vi "Read Mode Command.vi"   [LabVIEW 2023, in "Control Mode.lvclass"]
uses:
  Control Mode.lvclass
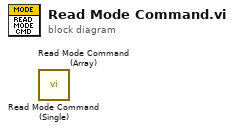
[diagram p0: block diagram]
diagram:
  n1 = call "Read Mode Command (Single).vi"() -> ()  [unwired: 8 in, 4 out]
  n2 = call "Read Mode Command (Array).vi"() -> ()  [unwired: 8 in, 4 out]
